vi "Region-det-ins-state-queue.vi"(8 "error in (no error)":errorcluster, 10 "State array":dbl[](array[numeric]), 11 "Plant state queue":refnum<queue>) -> (0 "error out":errorcluster)   [LabVIEW 2016]
uses:
  Plant_state.ctl
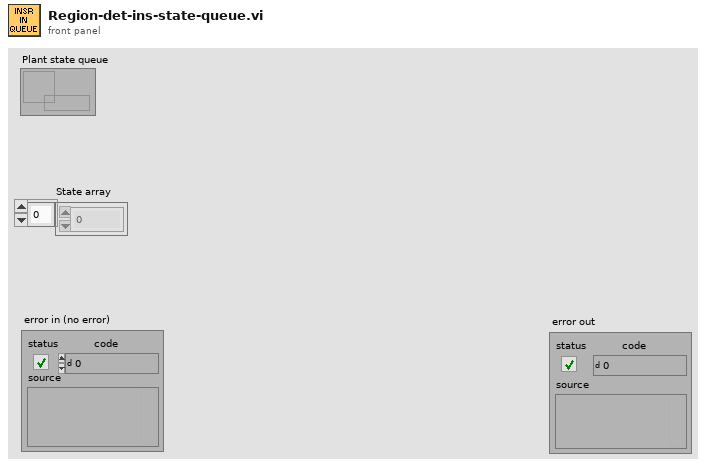
[diagram p1: front panel]
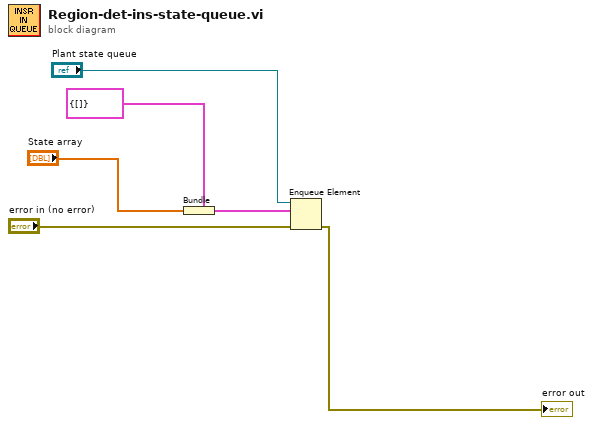
[diagram p0: block diagram]
diagram:
  n1 = Bundle(cluster=cluster{dbl[]} {[]}, "State array") -> (w3:cluster{dbl[]})
  n2 = Enqueue Element(queue="Plant state queue", element=w3, error in (no error)="error in (no error)") -> (error out=→"error out":errorcluster)  [unwired: 1 in, 2 out]
